vi "VS Errors_Inline Error Handler.vi"(8 "error in":errorcluster, 11 "Error Handling Cluster":T1) -> (0 "error out":errorcluster)   [LabVIEW 2013, in "CANOpen Addon Custom Device.lvlib"]
uses:
  CANOpen Addon Custom Device.lvlib
  _Controls/VS Errors_Error Handling Cluster.ctl
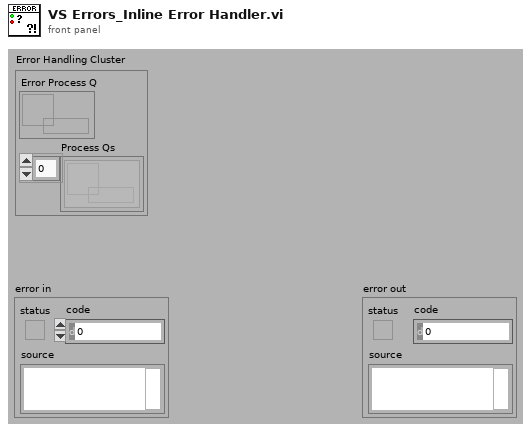
[diagram p1: front panel]
types:
  T1 = typedef "CANOpen Addon Custom Device.lvlib/VS Errors_Error Handling Cluster.ctl" = cluster{"Error Process Q":refnum<queue>, "Process Qs":refnum<queue>[]}
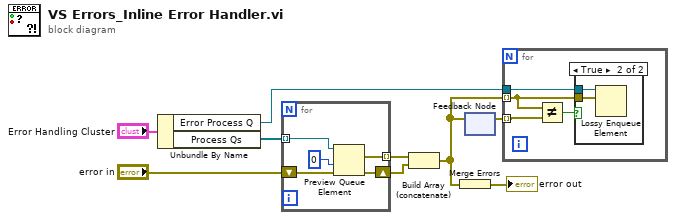
[diagram p0: block diagram]
diagram:
  n1 = Unbundle By Name("Error Handling Cluster") -> ("Error Process Q"=w2:refnum<queue>, "Process Qs"=w1:refnum<queue>[])
  n2 = for {
    tunnel: w1 -> [w13] mode=indexing
    shift-right: [w11] -> w6
    shift-left: "error in" -> [w14]
    tunnel: [w10] -> w7 mode=indexing
    n3 = Preview Queue Element(queue=w13, timeout in ms (-1)=0, error in (no error)=w14) -> (element=w10:errorcluster, error out=w11:errorcluster)  [unwired: 2 out]
  }
  n4 = Build Array (concatenate)(w7, w6) -> (w4:errorcluster[])
  n5 = Merge Errors(w4) -> (→"error out":errorcluster)
  n6 = feedback #1() -> (w5:errorcluster[])  [unwired: 1 in]
  n7 = feedback-in #1(w4) -> ()
  n8 = for {
    tunnel: w5 -> [w18] mode=indexing
    tunnel: w2 -> [w17]
    tunnel: w4 -> [w16] mode=indexing
    n9 = Not Equal?(x=w16, y=w18) -> (x != y?=w15:bool)
    n10 = case shown="True" w15 {
      tunnel: w17 -> [_ w20]
      tunnel: w16 -> [_ w19]
      frame False {
      }
      frame True {
        n11 = Lossy Enqueue Element(queue=w20, element=w19) -> ()  [unwired: 1 in, 4 out]
      }
    }
  }
